vi "quote and escape json string 2.vi"(9 "Is System Encoding (T)":bool=TRUE, 11 "base string":string) -> (3 "String out":string)   [LabVIEW 2024, in "JSONtext.lvlib"]
uses:
  JSONtext.lvlib
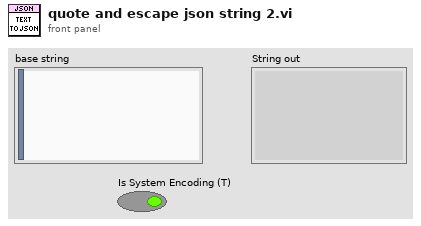
[diagram p1: front panel]
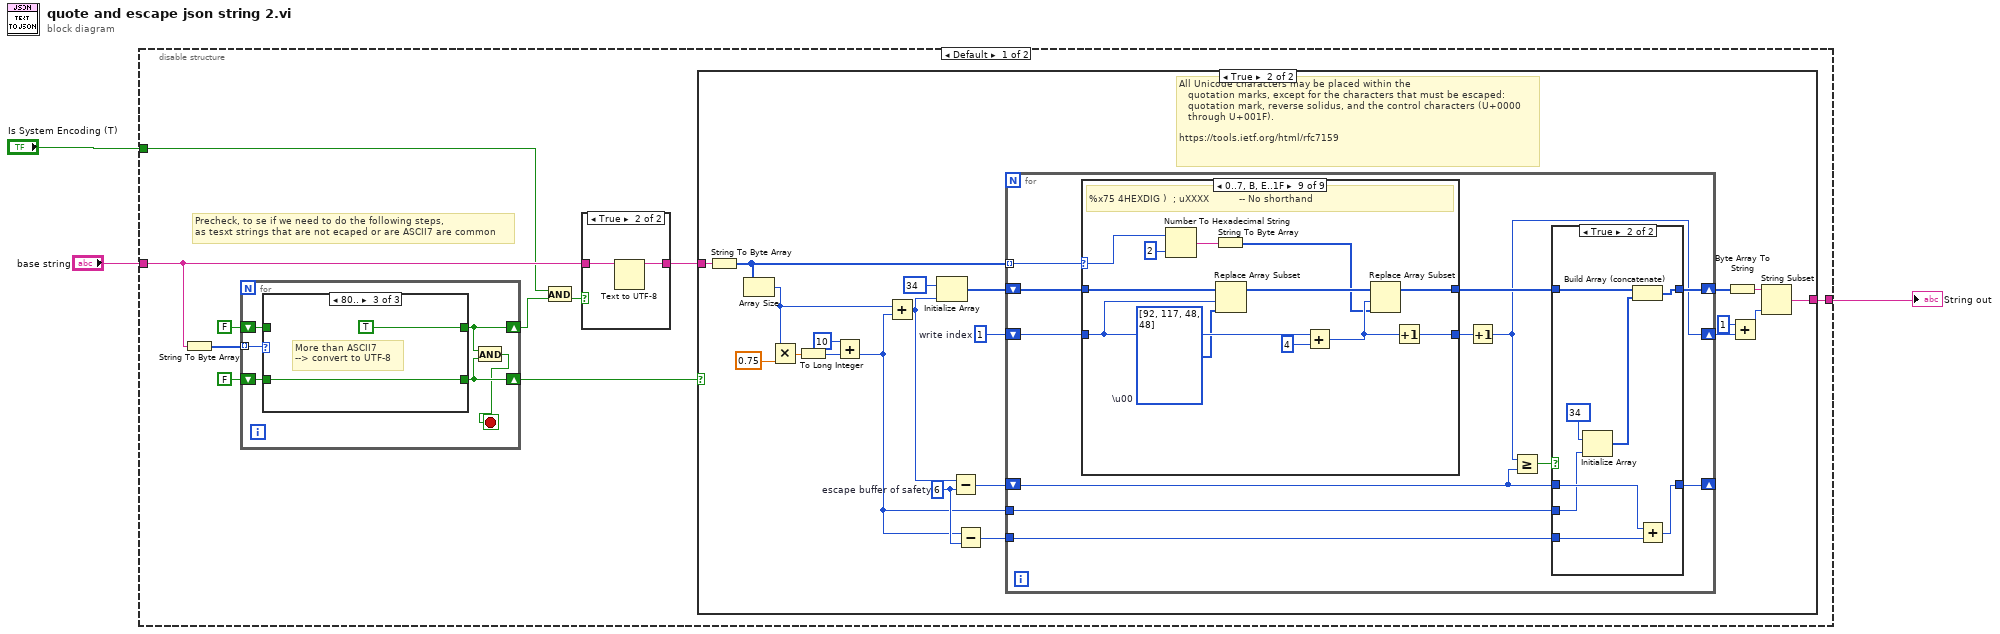
[diagram p0: block diagram]
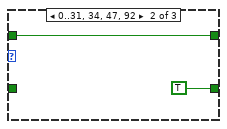
[diagram p4: hidden frame]
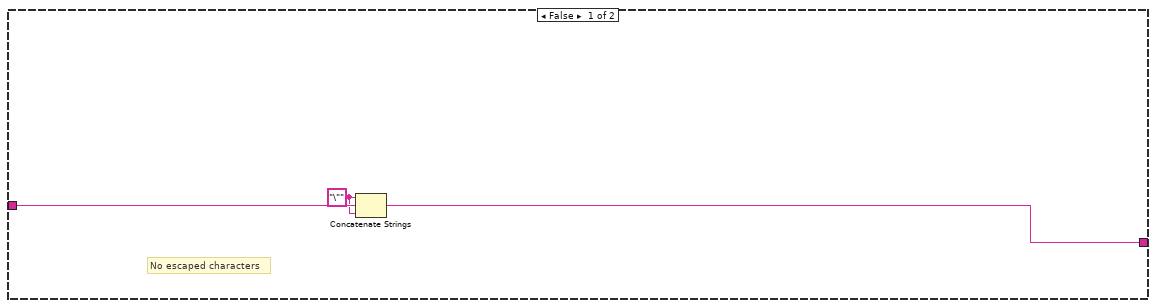
[diagram p5: hidden frame]
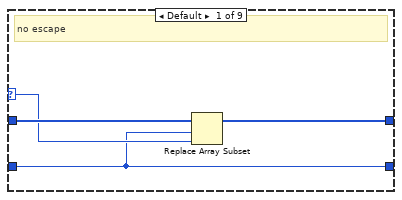
[diagram p7: hidden frame]
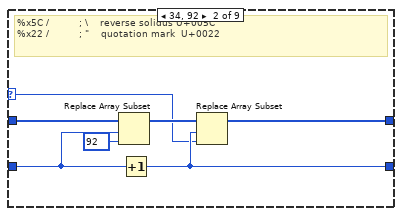
[diagram p8: hidden frame]
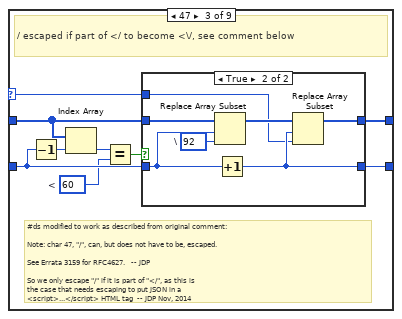
[diagram p9: hidden frame]
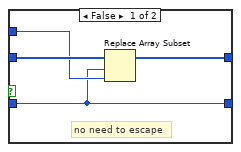
[diagram p10: hidden frame]
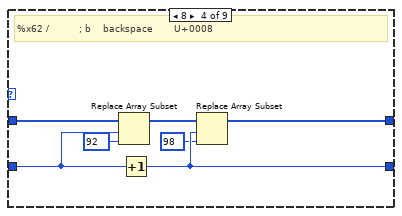
[diagram p11: hidden frame]
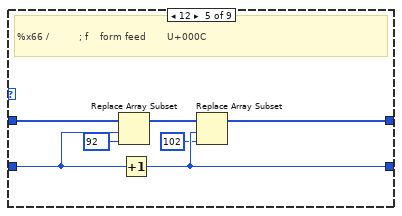
[diagram p12: hidden frame]
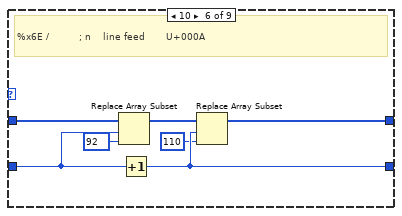
[diagram p13: hidden frame]
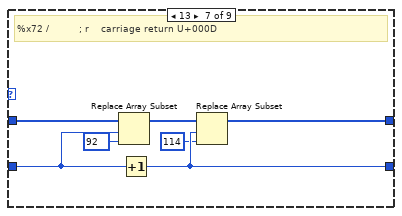
[diagram p14: hidden frame]
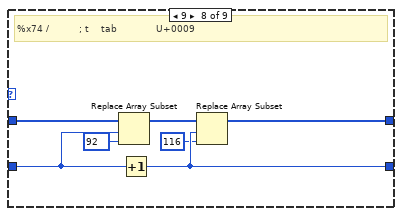
[diagram p15: hidden frame]
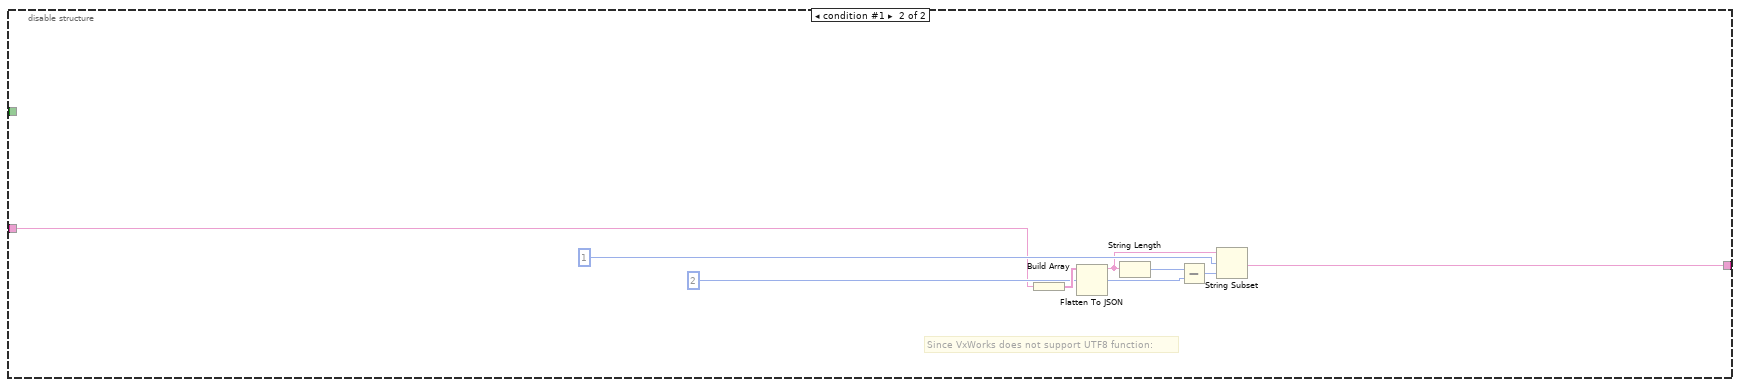
[diagram p16: hidden frame]
diagram:
  n1 = disable-structure shown="Default" {
    disable-tunnel: [w13 w154] -> w3
    disable-tunnel: "base string" -> [w11 w153]
    disable-tunnel: "Is System Encoding (T)" -> [w4 _]
    frame condition #0 (active) {
      # "Precheck, to se if we need to do the following steps,\nas tesxt strings that are not ecaped or are ASCII7 are common"
      n2 = String To Byte Array(string=w11) -> (unsigned byte array=w9:u8[])
      n3 = for {
        tunnel: w9 -> [w22] mode=indexing
        shift-right: [w21] -> w6
        shift-left: FALSE -> [w18]
        shift-right: [w20] -> w10
        shift-left: FALSE -> [w17]
        stop <- w19 stop-if-true
        n4 = case shown="80.." w22 {
          tunnel: [w24 w25 TRUE] -> w21
          tunnel: [w23 TRUE w27] -> w20
          tunnel: w18 -> [w24 w25 _]
          tunnel: w17 -> [w23 _ w27]
          frame Default {
          }
          frame 0..31, 34, 47, 92 {
          }
          frame 128.. {
            # "More than ASCII7\n--> convert to UTF-8"
          }
        }
        n5 = And(x=w21, y=w20) -> (x .and. y?=w19:bool)
      }
      n6 = And(x=w4, y=w6) -> (x .and. y?=w5:bool)
      n7 = case shown="True" w5 {
        tunnel: [w14 w16] -> w12
        tunnel: w11 -> [w14 w15]
        frame False {
        }
        frame True {
          n8 = Text to UTF-8(11:w15) -> (3:w16:string)  [unwired: 2 in, 1 out]
        }
      }
      n9 = case shown="True" w10 {
        tunnel: [w30 w52] -> w13
        tunnel: w12 -> [w31 w32]
        frame False {
          w29 = "\"" ("string")
          # "No escaped characters"
          n10 = Concatenate Strings(w29, w31, w29) -> (w30:string)
        }
        frame True {
          w38 = 6  # escape buffer of safety
          w50 = 1  # write index
          # "All Unicode characters may be placed within the\n   quotation marks, except for the characters that must be escaped:\n   quotation mark, reverse solidus, and the control characters (U+0000\n   through U+001F).\n\nhttps://tools.ietf.org/html/rfc7159"
          n11 = String To Byte Array(string=w32) -> (unsigned byte array=w44:u8[])
          n12 = Array Size(array=w44) -> (size(s)=w42:i32)
          n13 = Multiply(x=w42, y=0.75) -> (x*y=w45:dbl)
          n14 = To Long Integer(number=w45) -> (32bit integer=w39:i32)
          n15 = Add(x=10, y=w39) -> (x+y=w35:i32)
          n16 = Add(x=w42, y=w35) -> (x+y=w41:i32)
          n17 = Initialize Array(u8 34, w41) -> (w47:u8[])
          n18 = Subtract(x=w41, y=w38) -> (x-y=w40:i32)
          n19 = Subtract(x=w35, y=w38) -> (x-y=w37:i32)
          n20 = for {
            shift-right: [w61] -> w49
            shift-left: w47 -> [w64]
            shift-right: [w54] -> w43
            shift-left: w50 -> [w63]
            tunnel: w44 -> [w62] mode=indexing
            shift-right: [w58] -> _
            shift-left: w40 -> [w57]
            tunnel: w35 -> [w56]
            tunnel: w37 -> [w55]
            n21 = case shown="0..7, B, E..1F" w62 {
              selector: w62 -> [w76 w80 w92 _ _ _ _ _ w149]
              tunnel: w64 -> [w78 w85 w91 w112 w119 w126 w133 w140 w152]
              tunnel: [w77 w82 w94 w109 w116 w123 w130 w137 w151] -> w60
              tunnel: w63 -> [w75 w83 w90 w110 w117 w124 w131 w138 w150]
              tunnel: [w75 w81 w93 w108 w115 w122 w129 w136 w141] -> w59
              frame Default {
                # "no escape"
                n22 = Replace Array Subset(array=w78, new element=w76, index=w75) -> (w77:u8[])
              }
              frame 34, 92 {
                # "%x5C /          ; \\    reverse solidus U+005C\n%x22 /          ; \"    quotation mark  U+0022"
                n23 = Replace Array Subset(array=w85, new element=u8 92 ("new element/subarray"), index=w83) -> (w84:u8[])
                n24 = Increment(x=w83) -> (x+1=w81:i32)
                n25 = Replace Array Subset(array=w84, new element=w80, index=w81) -> (w82:u8[])
              }
              frame 47 {
                w86 = u8 60  # <
                # "#ds modified to work as described from original comment:\n\nNote: char 47, \"/\", can, but does not have to be, escaped.\n\nSee Errata 3159 for RFC4627.   -- JDP\n\nSo we only escape \"/\" if it is part of \"</\", as this is\nthe case that needs escaping to put JSON in a\n<script>...</script> HTML tag  -- JDP Nov, 2014"
                # "/ escaped if part of </ to become <\\/, see comment below"
                n26 = Decrement(x=w90) -> (x-1=w89:i32)
                n27 = Index Array(array=w91, index=w89) -> (element=w88:u8)
                n28 = Equal?(x=w88, y=w86) -> (x = y?=w87:bool)
                n29 = case shown="True" w87 {
                  tunnel: [w97 w104] -> w94
                  tunnel: [w95 w103] -> w93
                  tunnel: w92 -> [w96 w102]
                  tunnel: w91 -> [w98 w101]
                  tunnel: w90 -> [w95 w100]
                  frame False {
                    # "no need to escape"
                    n30 = Replace Array Subset(array=w98, new element=w96, index=w95) -> (w97:u8[])
                  }
                  frame True {
                    w99 = u8 92  # \
                    n31 = Replace Array Subset(array=w101, new element=w99, index=w100) -> (w105:u8[])
                    n32 = Increment(x=w100) -> (x+1=w103:i32)
                    n33 = Replace Array Subset(array=w105, new element=w102, index=w103) -> (w104:u8[])
                  }
                }
              }
              frame 8 {
                # "%x62 /          ; b    backspace       U+0008"
                n34 = Replace Array Subset(array=w112, new element=u8 92 ("new element/subarray"), index=w110) -> (w111:u8[])
                n35 = Increment(x=w110) -> (x+1=w108:i32)
                n36 = Replace Array Subset(array=w111, new element=u8 98 ("new element/subarray"), index=w108) -> (w109:u8[])
              }
              frame 12 {
                # "%x66 /          ; f    form feed       U+000C"
                n37 = Replace Array Subset(array=w119, new element=u8 92 ("new element/subarray"), index=w117) -> (w118:u8[])
                n38 = Increment(x=w117) -> (x+1=w115:i32)
                n39 = Replace Array Subset(array=w118, new element=u8 102 ("new element/subarray"), index=w115) -> (w116:u8[])
              }
              frame 10 {
                # "%x6E /          ; n    line feed       U+000A"
                n40 = Replace Array Subset(array=w126, new element=u8 92 ("new element/subarray"), index=w124) -> (w125:u8[])
                n41 = Increment(x=w124) -> (x+1=w122:i32)
                n42 = Replace Array Subset(array=w125, new element=u8 110 ("new element/subarray"), index=w122) -> (w123:u8[])
              }
              frame 13 {
                # "%x72 /          ; r    carriage return U+000D"
                n43 = Replace Array Subset(array=w133, new element=u8 92 ("new element/subarray"), index=w131) -> (w132:u8[])
                n44 = Increment(x=w131) -> (x+1=w129:i32)
                n45 = Replace Array Subset(array=w132, new element=u8 114 ("new element/subarray"), index=w129) -> (w130:u8[])
              }
              frame 9 {
                # "%x74 /          ; t    tab             U+0009"
                n46 = Replace Array Subset(array=w140, new element=u8 92 ("new element/subarray"), index=w138) -> (w139:u8[])
                n47 = Increment(x=w138) -> (x+1=w136:i32)
                n48 = Replace Array Subset(array=w139, new element=u8 116 ("new element/subarray"), index=w136) -> (w137:u8[])
              }
              frame 0..7, 11, 14..31 {
                w142 = u8[] [92, 117, 48, 48]  # \u00
                # "%x75 4HEXDIG )  ; uXXXX          -- No shorthand"
                n49 = Number To Hexadecimal String(1:i16 2 ("width (-)"), 2:w149) -> (0:w144:string)
                n50 = String To Byte Array(string=w144) -> (unsigned byte array=w146:u8[])
                n51 = Replace Array Subset(array=w152, new element=w142, index=w150) -> (w148:u8[])
                n52 = Add(x=w150, y=4) -> (x+y=w147:i32)
                n53 = Replace Array Subset(array=w148, new element=w146, index=w147) -> (w151:u8[])
                n54 = Increment(x=w147) -> (x+1=w141:i32)
              }
            }
            n55 = Increment(x=w59) -> (x+1=w54:i32)
            n56 = Greater Or Equal?(x=w54, y=w57) -> (x >= y?=w53:bool)
            n57 = case shown="True" w53 {
              tunnel: [w66 w69] -> w61
              tunnel: w60 -> [w66 w70]
              tunnel: [w65 w72] -> w58
              tunnel: w57 -> [w65 w73]
              tunnel: w56 -> [_ w71]
              tunnel: w55 -> [_ w74]
              frame False {
              }
              frame True {
                n58 = Initialize Array(u8 34, w71) -> (w68:u8[])
                n59 = Build Array (concatenate)(w70, w68) -> (w69:u8[])
                n60 = Add(x=w73, y=w74) -> (x+y=w72:i32)
              }
            }
          }
          n61 = Byte Array To String(unsigned byte array=w49) -> (string=w51:string)
          n62 = Add(x=1, y=w43) -> (x+y=w36:i32)
          n63 = String Subset(string=w51, length (rest)=w36) -> (substring=w52:string)  [unwired: 1 in]
        }
      }
    }
    frame condition #1 {
      # "Since VxWorks does not support UTF8 function:"
      n64 = Build Array(w153) -> (w160:string[])
      n65 = Flatten To JSON(anything=w160) -> (JSON string=w157:string)  [unwired: 2 in, 1 out]
      n66 = String Length(string=w157) -> (length=w158:i32)
      n67 = Subtract(x=w158, y=2 ("x")) -> (x-y=w156:i32)
      n68 = String Subset(string=w157, offset (0)=1, length (rest)=w156) -> (substring=w154:string)
    }
  }
  "String out" <- w3
